vi "Set Password.vi"(8 "error in (no error)":errorcluster, 9 "New password":string, 10 "ProjectItem Refnum":refnum<vi>, 11 "SDIST in":refnum<class "NI_AB_API_DSDIST.lvclass">) -> (0 "error out":errorcluster, 3 "SDIST out":refnum<class "NI_AB_API_DSDIST.lvclass">)   [LabVIEW 2020, in "NI_AB_API_DSDIST.lvclass"]
uses:
  <vilib>/AppBuilder/AB_API/DSDIST/NI_AB_API_DSDIST.lvclass
  <vilib>/AppBuilder/AB_API/SDIST/NI_AB_API_SDIST.lvclass
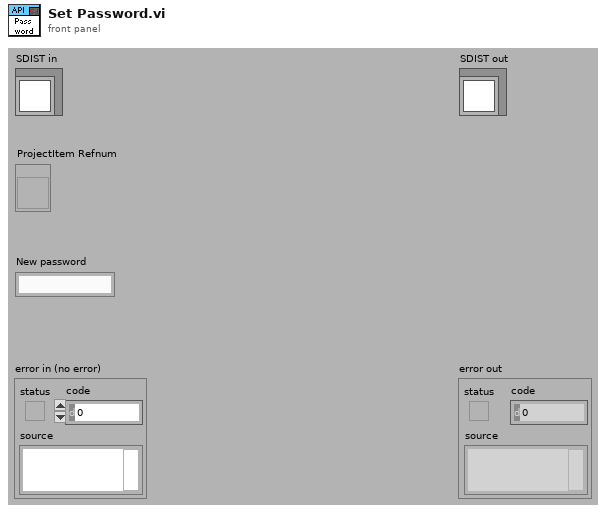
[diagram p1: front panel]
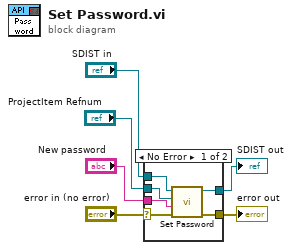
[diagram p0: block diagram]
diagram:
  n1 = case shown="No Error" "error in (no error)" {
    selector: "error in (no error)" -> [w9 w14]
    tunnel: [w8 w14] -> w5
    tunnel: [w7 w13] -> w3
    tunnel: "SDIST in" -> [w12 w13]
    tunnel: "ProjectItem Refnum" -> [w11 _]
    tunnel: "New password" -> [w10 _]
    frame No Error {
      n2 = call-parent "Set Password.vi"("error in (no error)"=w9, "New password"=w10, "ProjectItem Refnum"=w11, "SDIST in"=w12) -> ("error out"=w8:errorcluster, "SDIST out"=w7:refnum<class "NI_AB_API_DSDIST.lvclass">)  [unwired: 6 in]
    }
    frame Error {
    }
  }
  "error out" <- w5
  "SDIST out" <- w3
